vi "PROCURA_CONTROLE.vi"(8 "error in":errorcluster, 10 "name":string, 11 "Controls in":refnum<vi>[](array[refnum])) -> (0 "error out":errorcluster, 3 "element":refnum<vi>)   [LabVIEW 2019]
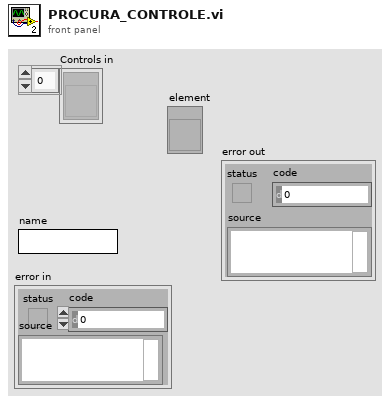
[diagram p1: front panel]
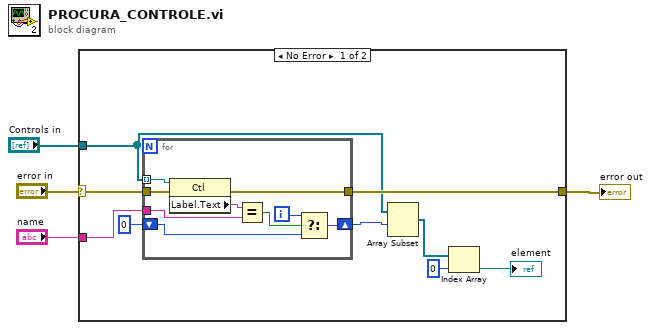
[diagram p0: block diagram]
diagram:
  n1 = case shown="No Error" "error in" {
    selector: "error in" -> [w11 w23]
    tunnel: [w13 w23] -> w4
    tunnel: "name" -> [w12 _]
    tunnel: "Controls in" -> [w9 _]
    frame No Error {
      n2 = for {
        tunnel: w9 -> [w22] mode=indexing
        tunnel: w12 -> [w20]
        shift-right: [w17] -> w8
        shift-left: 0 -> [w16]
        tunnel: w11 -> [w15]
        tunnel: [w14] -> w13
        i -> [w18]
        n3 = property class="Ctl"(reference=w22, error in=w15) -> (error out=w14:errorcluster, "Label.Text"=w21:string)  [unwired: 1 out]
        n4 = Equal?(x=w21, y=w20) -> (x = y?=w19:bool)
        n5 = Select(t=w18, s=w19, f=w16) -> (s? t:f=w17:i32)
      }
      n6 = Array Subset(array=w9, index=w8) -> (w7:refnum<vi>[])  [unwired: 1 in]
      n7 = Index Array(array=w7, index=0) -> (element=→"element":refnum<vi>)
    }
    frame Error {
    }
  }
  "error out" <- w4
